vi "Copy Config Converter.vi"(8 "error in (no error)":errorcluster) -> (0 "error out":errorcluster)   [LabVIEW 2015, in "AIT 429 System Explorer.lvlib"]
uses:
  <vilib>/Utility/sysdir.llb/System Directory Type.ctl
  AIT 429 System Explorer.lvlib
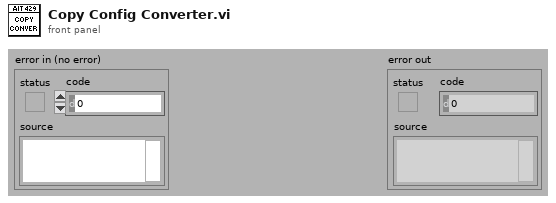
[diagram p1: front panel]
types:
  T1 = typedef "System Directory Type.ctl" = i32
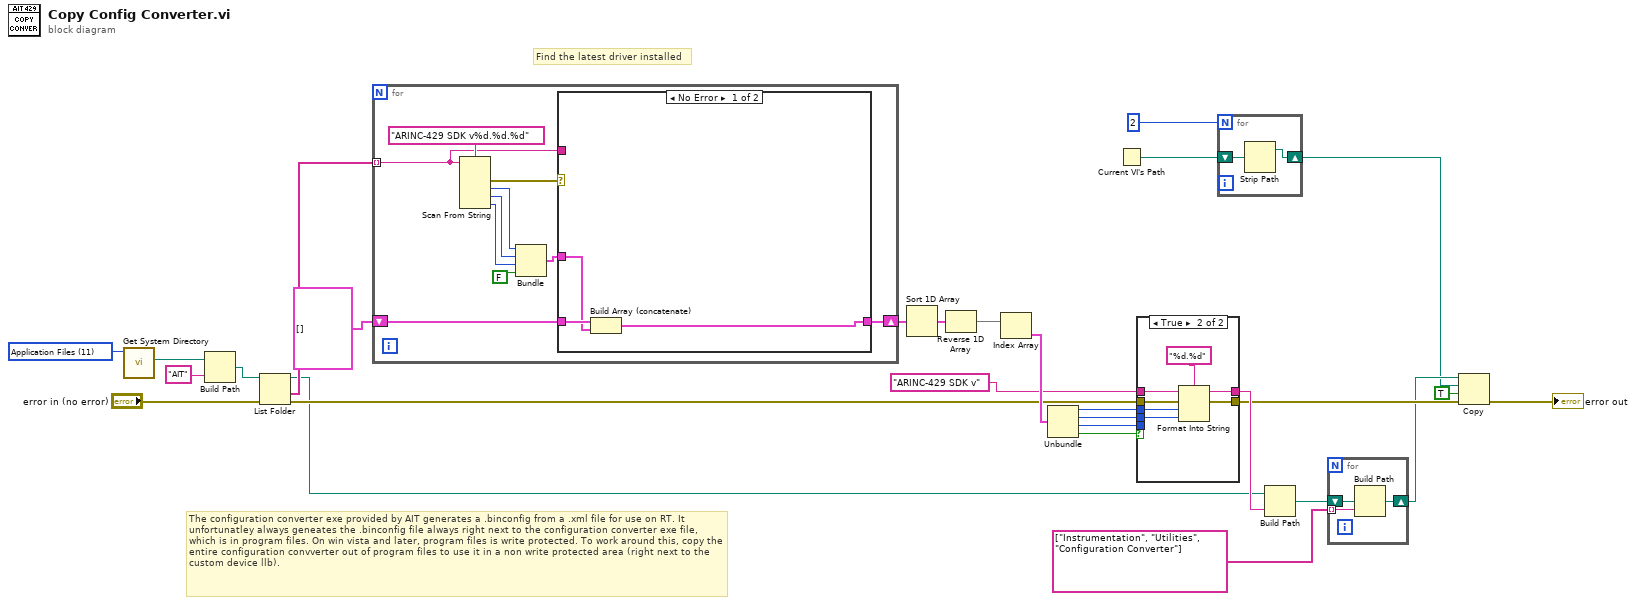
[diagram p0: block diagram]
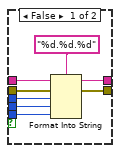
[diagram p2: hidden frame]
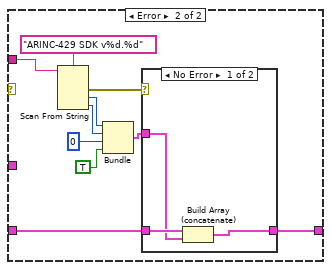
[diagram p3: hidden frame]
diagram:
  w28 = T1 11 items=["User Home"=0, "User Desktop"=1, "User Documents"=2, "User Application Data"=3, "User Preferences"=4, "User Temporary"=5, "Public Documents"=6, "Public Application Data"=7, "Public Preferences"=8, "Public Cache"=13, "System Core Libraries"=9, "System Installed Libraries"=10, "Application Files"=11, "Boot Volume Root"=12] ("system directory type")
  # "The configuration converter exe provided by AIT generates a .binconfig from a .xml file for use on RT. It unfortunatley always geneates the .binconfig file always right next to the configuration converter exe file, which is in program files. On win vista and later, program files is write protected. To work around this, copy the entire configuration convverter out of program files to use it in a non write protected area (right next to the custom device llb)."
  # "Find the latest driver installed"
  n1 = call <vilib>:"Get System Directory.vi"("system directory type"=w28) -> ("system directory"=w27:path)  [unwired: 10 in]
  n2 = Build Path(base path=w27, name or relative path="AIT") -> (appended path=w25:path)
  n3 = List Folder(path=w25, error in="error in (no error)") -> (path out=w11:path, folder names=w23:string[], error out=w17:errorcluster)  [unwired: 2 in, 1 out]
  n4 = for {
    tunnel: w23 -> [w30] mode=indexing
    shift-right: [w31] -> w15
    shift-left: cluster{i32, i32, i32, bool}[] [] -> [w33]
    n5 = Scan From String(format string="ARINC-429 SDK v%d.%d.%d", input string=w30) -> (error out=w34:errorcluster, output 1=w36:i32, output 2=w35:i32, output 3=w38:i32)  [unwired: 5 in, 2 out]
    n6 = Bundle(w36, w35, w38, FALSE) -> (w32:cluster{i32, i32, i32, bool})  [unwired: 1 in]
    n7 = case shown="No Error" w34 {
      tunnel: w33 -> [w41 w45]
      tunnel: w32 -> [w40 _]
      tunnel: [w39 w43] -> w31
      tunnel: w30 -> [_ w50]
      frame No Error {
        n8 = Build Array (concatenate)(w41, w40) -> (w39:cluster{i32, i32, i32, bool}[])
      }
      frame Error {
        n9 = Scan From String(format string="ARINC-429 SDK v%d.%d", input string=w50) -> (error out=w49:errorcluster, output 1=w48:i32, output 2=w47:i32)  [unwired: 4 in, 2 out]
        n10 = Bundle(w48, w47, 0, TRUE) -> (w44:cluster{i32, i32, i32, bool})  [unwired: 1 in]
        n11 = case shown="No Error" w49 {
          tunnel: w45 -> [w54 w55]
          tunnel: w44 -> [w53 _]
          tunnel: [w52 w55] -> w43
          frame No Error {
            n12 = Build Array (concatenate)(w54, w53) -> (w52:cluster{i32, i32, i32, bool}[])
          }
          frame Error {
          }
        }
      }
    }
  }
  n13 = Sort 1D Array(array=w15) -> (sorted array=w22:cluster{i32, i32, i32, bool}[])
  n14 = Reverse 1D Array(array=w22) -> (reversed array=w14:cluster{i32, i32, i32, bool}[])
  n15 = Index Array(array=w14) -> (element=w21:cluster{i32, i32, i32, bool})  [unwired: 1 in]
  n16 = Unbundle(w21) -> (w20:i32, w19:i32, w18:i32, w2:bool)
  n17 = Current VI's Path() -> (path=w6:path)
  n18 = case shown="True" w2 {
    tunnel: w20 -> [w62 w69]
    tunnel: w19 -> [w61 w68]
    tunnel: w18 -> [w60 _]
    tunnel: w17 -> [w59 w67]
    tunnel: "ARINC-429 SDK v" ("format string") -> [w58 w66]
    tunnel: [w57 w65] -> w12
    tunnel: [w56 w64] -> w8
    frame False {
      n19 = Format Into String(format string="%d.%d.%d", initial string=w58, error in=w59, w62, w61, w60) -> (resulting string=w57:string, error out=w56:errorcluster)
    }
    frame True {
      n20 = Format Into String(format string="%d.%d", initial string=w66, error in=w67, w69, w68) -> (resulting string=w65:string, error out=w64:errorcluster)
    }
  }
  n21 = for {
    N: 2 -> [_]
    shift-right: [w71] -> w4
    shift-left: w6 -> [w72]
    n22 = Strip Path(path=w72) -> (stripped path=w71:path)  [unwired: 1 out]
  }
  n23 = Build Path(base path=w11, name or relative path=w12) -> (appended path=w10:path)
  n24 = for {
    tunnel: string[] ["Instrumentation", "Utilities", "Configuration Converter"] -> [w74] mode=indexing
    shift-right: [w73] -> w7
    shift-left: w10 -> [w75]
    n25 = Build Path(base path=w75, name or relative path=w74) -> (appended path=w73:path)
  }
  n26 = Copy(8:w8, 9:TRUE ("overwrite (F)"), 10:w4, 11:w7) -> (0:→"error out":errorcluster)  [unwired: 1 in, 2 out]
